vi "Decode Scan Data.vi"(8 "error in (no error)":errorcluster, 11 "Packet Data In":string) -> (0 "error IO":errorcluster, 2 "Distance":u32[](array[numeric]) format="%08d", 3 "Packet Header":T1 {"Scan Number" format="%04d"; "Status Flags" format="%04x"; "Timestamp Sync" format="%016x"; "Timestamp Raw" format="%016x"; "Packet Number" format="%04d"; "Header Size" format="%04d"; "Packet Size" format="%04x"; "Packet Type" format="%04x"})   [LabVIEW 2019, in "PF_API.lvclass"]
uses:
  PF_API.lvclass
  Packet Structure A.ctl
panel:
  out "length":i32
  out "Magic Byte":u16 format="%x"
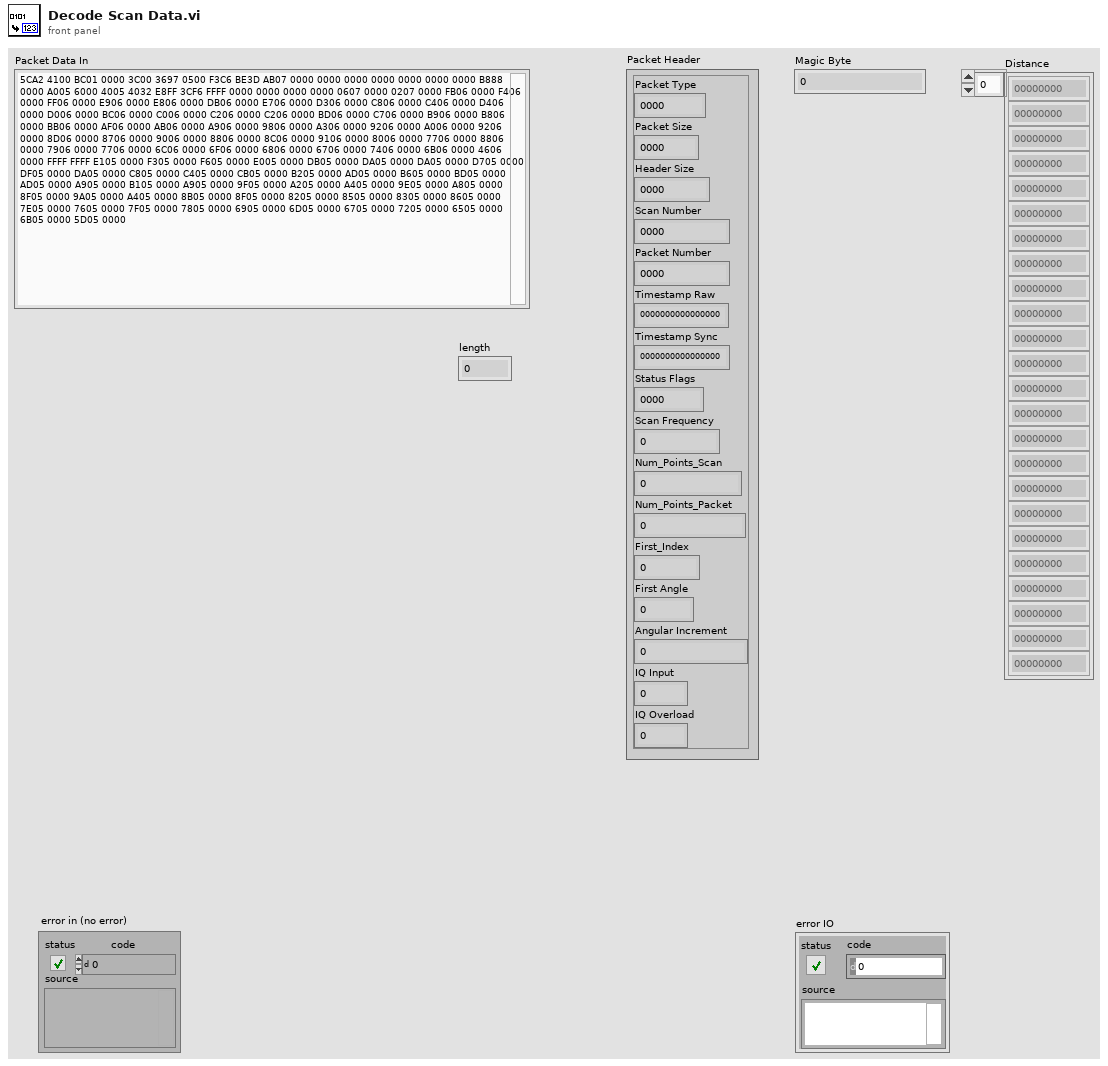
[diagram p1: front panel]
types:
  T1 = typedef "Packet Structure A.ctl" = cluster{"Packet Type":u16, "Packet Size":u32, "Header Size":u16, "Scan Number":u16, "Packet Number":u16, "Timestamp Raw":u64, "Timestamp Sync":u64, "Status Flags":u32, "Scan Frequency":u32, "Num_Points_Scan":u16, "Num_Points_Packet":u16, "First_Index":u16, "First Angle":i32, "Angular Increment":i32, "IQ Input":u32, "IQ Overload":u32}
  T2 = enum16{"big-endian, network order", "native, host order", "little-endian"}
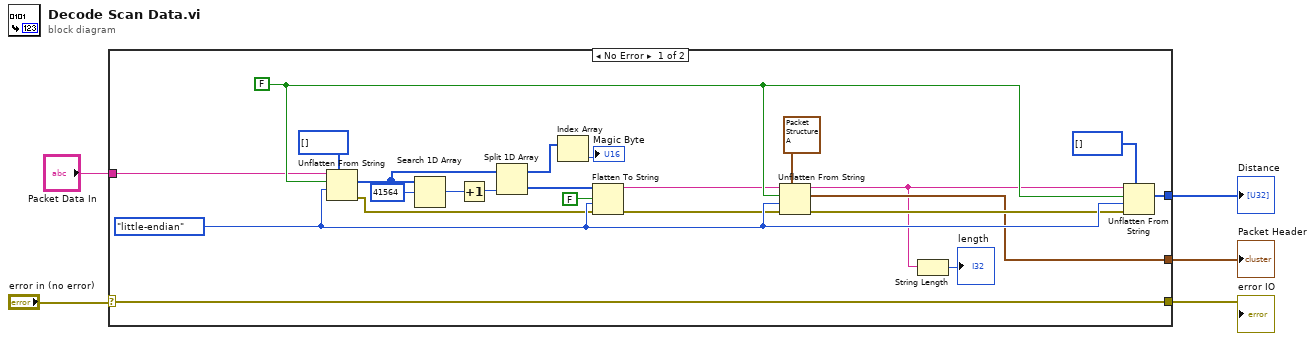
[diagram p0: block diagram]
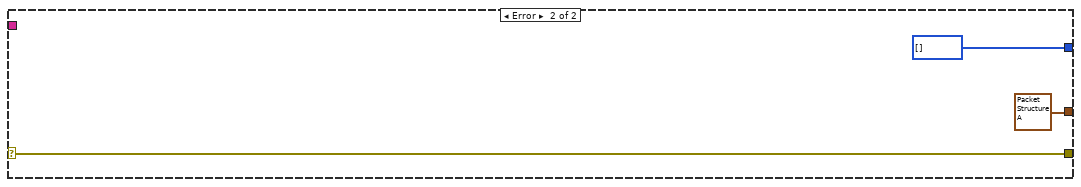
[diagram p2: hidden frame]
diagram:
  n1 = case shown="No Error" "error in (no error)" {
    selector: "error in (no error)" -> [w10 w29]
    tunnel: [w25 T1 {"Packet Type"=0, "Packet Size"=0, "Header Size"=0, "Scan Number"=0, "Packet Number"=0, "Timestamp Raw"=0, "Timestamp Sync"=0, "Status Flags"=0, "Scan Frequency"=0, "Num_Points_Scan"=0, "Num_Points_Packet"=0, "First_Index"=0, "First Angle"=0, "Angular Increment"=0, "IQ Input"=0, "IQ Overload"=0} ("Packet A")] -> w5
    tunnel: "Packet Data In" -> [w24 _]
    tunnel: [w22 u32[] []] -> w3
    tunnel: [w10 w29] -> w1
    frame No Error {
      w26 = FALSE ("data includes array or string size? (T)")
      w28 = T2."little-endian" ("byte order (0:big-endian, network order)")
      n2 = Unflatten From String(type=u16[] [], binary string=w24, data includes array or string size? (T)=w26, byte order (0:big-endian, network order)=w28) -> (value=w13:u16[], error out=w14:errorcluster)  [unwired: 1 in, 1 out]
      n3 = Search 1D Array(1D array=w13, element=u16 41564) -> (index of element=w20:i32)  [unwired: 1 in]
      n4 = Increment(x=w20) -> (x+1=w21:i32)
      n5 = Split 1D Array(array=w13, index=w21) -> (first subarray=w12:u16[], second subarray=w17:u16[])
      n6 = Index Array(array=w12) -> (element=→"Magic Byte":u16)  [unwired: 1 in]
      n7 = Flatten To String(anything=w17, prepend array or string size? (T)=FALSE, byte order (0:big-endian, network order)=w28, error in (no error)=w14) -> (data string=w9:string, error out=w15:errorcluster)  [unwired: 1 out]
      n8 = Unflatten From String(type=T1 {"Packet Type"=0, "Packet Size"=0, "Header Size"=0, "Scan Number"=0, "Packet Number"=0, "Timestamp Raw"=0, "Timestamp Sync"=0, "Status Flags"=0, "Scan Frequency"=0, "Num_Points_Scan"=0, "Num_Points_Packet"=0, "First_Index"=0, "First Angle"=0, "Angular Increment"=0, "IQ Input"=0, "IQ Overload"=0} ("Packet A"), binary string=w9, data includes array or string size? (T)=w26, byte order (0:big-endian, network order)=w28, error in (no error)=w15) -> (rest of the binary string=w7:string, value=w25:T1, error out=w27:errorcluster)
      n9 = String Length(string=w7) -> (length=→"length":i32)
      n10 = Unflatten From String(type=u32[] [], binary string=w7, data includes array or string size? (T)=w26, byte order (0:big-endian, network order)=w28, error in (no error)=w27) -> (value=w22:u32[])  [unwired: 2 out]
    }
    frame Error {
    }
  }
  "Packet Header" <- w5
  "Distance" <- w3
  "error IO" <- w1
